vi "Instrument.DAQ.TestLauncher.vi"() -> ()   [LabVIEW 2019, in "Instrument.Lockin.lvlib" / "Instrument.DAQ.lvclass"]
uses:
  Instrument.DAQ.lvclass
  <vilib>/JKI/JKI SMO/SMO/Typedefs/SMOState --Enum.ctl
  Typedefs/AO.Channel--Cluster--Array.ctl
  Typedefs/AO.Channel--Cluster.ctl
  Typedefs/AO.Channel.Function--Enum.ctl
  Typedefs/REF.Channel--Cluster--Array.ctl
  Typedefs/REF.Channel--Cluster.ctl
  Typedefs/DAQ.Sampling.Sampling--Cluster.ctl
  Typedefs/Channel.Gain--Cluster--Array.ctl
  Typedefs/Channel.Gain--Cluster.ctl
  Typedefs/Status--enum.ctl
  Typedefs/DAQ.Configuration--Cluster.ctl
  Typedefs/DAQ.Config.AO.Range--enum.ctl
  Typedefs/DAQ.TerminalConfiguration--ring.ctl
  Typedefs/DAQ.Config.AI.Range--enum.ctl
  Typedefs/DAQ.Config.AI.Coupling--enum.ctl
  C:/Program Files/National Instruments/LabVIEW 2019/vi.lib/JKI/JKI SMO/SMO/SMO.lvclass
  <vilib>/JKI/JKI SMO/SMO/SMO.lvclass/SMO.ctl
  Typedefs/State--enum.ctl
  Typedefs/DAQ.Sampling--Cluster.ctl
  Instrument.Lockin/Typedefs/Results Type--Enum.ctl
  <vilib>/JKI/JKI SMO/SMO/Private/ReftoDVR--SMO.vi
  Instrument.Lockin/Instrument.Lockin.lvclass
  <vilib>/JKI/JKI SMO/SMO/SMO.lvclass
panel:
  out "DAQ state":T1
  in  "Tab Control 2":T2(tab)
  out "AO":waveform(dbl)[](graph)=[{"t0"=timestamp(3826459409.893437 s since 1904-01-01), "dt"=4.8830747732362694e-06, "Y"=array[15753 elements], "attributes"=variant("AO Channel"=variant(i32 1))}, {"t0"=timestamp(3826459409.893437 s since 1904-01-01), "dt"=4.8830747732362694e-06, "Y"=array[15753 elements], "attributes"=variant("AO Channel"=variant(i32 2))}, {"t0"=timestamp(3826459409.893437 s since 1904-01-01), "dt"=4.8830747732362694e-06, "Y"=array[15753 elements], "attributes"=variant("AO Channel"=variant(i32 3))}, {"t0"=timestamp(3826459409.893437 s since 1904-01-01), "dt"=4.8830747732362694e-06, "Y"=array[15753 elements], "attributes"=variant("AO Channel"=variant(i32 4))}]
  out "AI":waveform(dbl)[](graph)=[{"t0"=timestamp(3826459409.8699865 s since 1904-01-01), "dt"=4.883074773236228e-06, "Y"=array[15753 elements], "attributes"=variant("AI Channel"=variant(i32 1), "NI_ChannelName"=variant(string "PXI1Slot2/ai0"), "NI_UnitDescription"=variant(string "Volts"))}, {"t0"=timestamp(3826459409.8699865 s since 1904-01-01), "dt"=4.883074773236228e-06, "Y"=array[15753 elements], "attributes"=variant("AI Channel"=variant(i32 2), "NI_ChannelName"=variant(string "PXI1Slot2/ai1"), "NI_UnitDescription"=variant(string "Volts"))}, {"t0"=timestamp(3826459409.860074 s since 1904-01-01), "dt"=4.883074773236228e-06, "Y"=array[15753 elements], "attributes"=variant("AI Channel"=variant(i32 3), "NI_ChannelName"=variant(string "PXI1Slot3/ai0"), "NI_UnitDescription"=variant(string "Volts"))}, {"t0"=timestamp(3826459409.860074 s since 1904-01-01), "dt"=4.883074773236228e-06, "Y"=array[15753 elements], "attributes"=variant("AI Channel"=variant(i32 4), "NI_ChannelName"=variant(string "PXI1Slot3/ai1"), "NI_UnitDescription"=variant(string "Volts"))}]
  out "WFM 3":waveform(dbl)[](graph)=[{"t0"=timestamp(3826459409.893437 s since 1904-01-01), "dt"=4.8830747732362694e-06, "Y"=array[15753 elements], "attributes"=variant("AO Channel"=variant(i32 1))}, {"t0"=timestamp(3826459409.893437 s since 1904-01-01), "dt"=4.8830747732362694e-06, "Y"=array[15753 elements], "attributes"=variant("Reference Channel"=variant(i32 1))}, {"t0"=timestamp(3826459409.8699865 s since 1904-01-01), "dt"=4.883074773236228e-06, "Y"=array[15753 elements], "attributes"=variant("AI Channel"=variant(i32 1), "NI_ChannelName"=variant(string "PXI1Slot2/ai0"), "NI_UnitDescription"=variant(string "Volts"))}]
  out "REF":waveform(dbl)[](graph)=[{"t0"=timestamp(3826459409.893437 s since 1904-01-01), "dt"=4.8830747732362694e-06, "Y"=array[15753 elements], "attributes"=variant("Reference Channel"=variant(i32 1))}, {"t0"=timestamp(3826459409.893437 s since 1904-01-01), "dt"=4.8830747732362694e-06, "Y"=array[15753 elements], "attributes"=variant("Reference Channel"=variant(i32 1))}]
  out "Results":dbl[](graph)
  in  "Reset DAQ":bool
  in  "Stop DAQ":bool
  in  "Start DAQ":bool
  in  "Tab Control":enum32{"Output", "REF", "DAQ"}(tab)=enum."DAQ"
  in  "Channels: AO":T3=[{"Enable?"=TRUE, "Channel"=0, "Amplitude"=0.1, "Offset"=0.0, "Frequency"=15.0, "Phase"=0.0, "Function"=enum."sine", "Sweeping?"=FALSE, "Limit AC"=FALSE, "Limit DC?"=FALSE, "Duty Cycle"=FALSE}, {"Enable?"=TRUE, "Channel"=0, "Amplitude"=0.05, "Offset"=0.0, "Frequency"=13.0, "Phase"=0.0, "Function"=enum."sine", "Sweeping?"=FALSE, "Limit AC"=FALSE, "Limit DC?"=FALSE, "Duty Cycle"=FALSE}] {"Phase" format="%#_3g"; "Frequency" min=0.0001 max=200000.0 format="%#_6p"; "Offset" format="%#_6p"; "Amplitude" min=0.0 max=10.0 format="%#_6p"}
  in  "Channels: Lockin":T6=[{"Enable?"=TRUE, "Channel"=1, "Frequency"=13.0, "Phase"=0.0, "TC"=1e-05, "Roll-Off"=1}] {"Roll-Off" min=1 max=4; "TC" min=1e-06 max=100.0 format="%#_3p"; "Phase" format="%#_3p"; "Frequency" min=1e-06 max=102400.0 format="%#_6p"; "Channel" min=1}
  in  "Gain":T8
  in  "sampling":T10={"Fs"=204789.0, "#s"=15753} {"Fs" format="%#_13g"}
  in  "New Ch []":T11[](array[typedef])=[{"Device"="PXI1Slot2", "Lockin.AO"="", "AO.Ch"="", "AO.Range"=enum."±0.1", "AO terminal config"=0, "Lockin.AI"="", "AI.Ch"="", "AI.Range"=enum."±0.316", "AI.Coupling"=10050, "AI terminal config"=0}, {"Device"="PXI1Slot3", "Lockin.AO"="", "AO.Ch"="", "AO.Range"=enum."±0.1", "AO terminal config"=0, "Lockin.AI"="", "AI.Ch"="", "AI.Range"=enum."±0.316", "AI.Coupling"=10050, "AI terminal config"=0}] {"AI terminal config" items=[""=-1, "differential"=10106, "pseudodifferential"=12529]; "AI.Coupling" items=[""=0, "AC"=10045, "DC"=10050, "GND"=10066]; "AO terminal config" items=[""=-1, "differential"=10106, "pseudodifferential"=12529]}
  out "SMO State":T16=enum."Stopped"
  out "error out":errorcluster
  in  "Stop":bool
  # "Basic SMO Test Launcher"
  # "For instructions on how to use the JKI State Machine Objects, examples and video tutorials, visit:\nhttp://jki.net/state-machine-objects/\n\nJKI State Machine Objects™\nhttp://jki.net/state-machine-objects/\nCopyright (C) 2005-2015, JKI <info@jki.net>\nALL RIGHTS RESERVED"
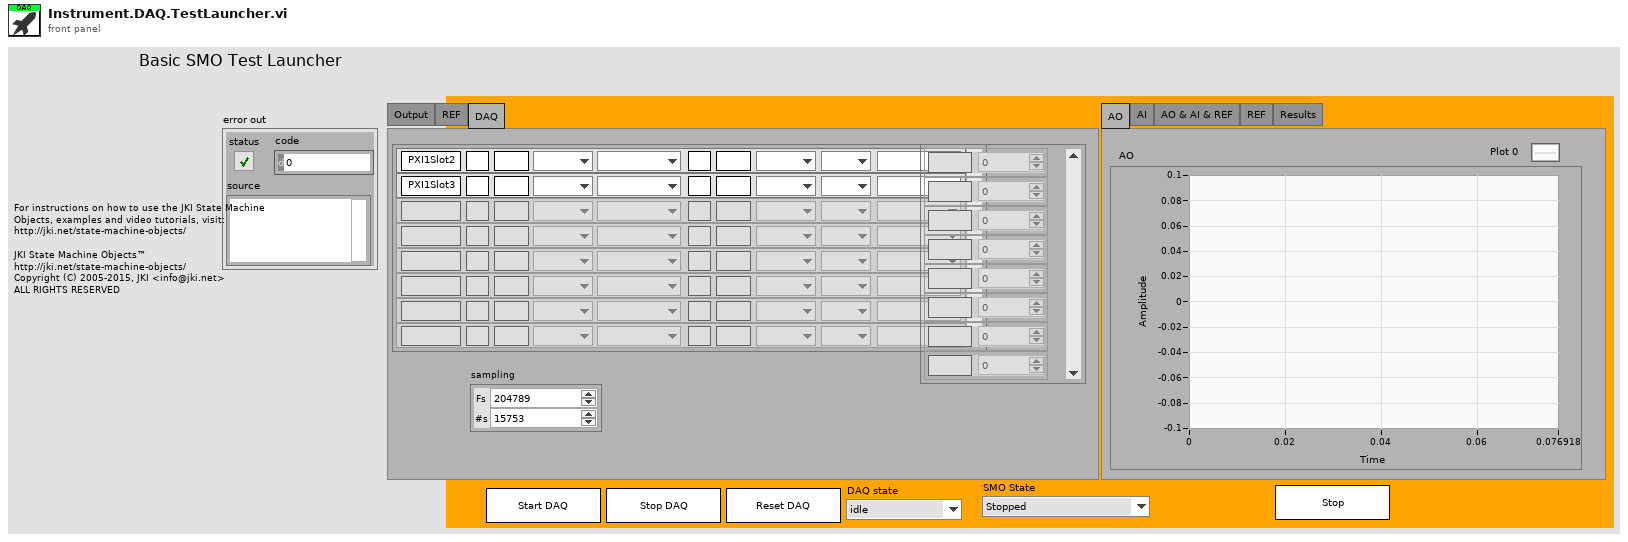
[diagram p1: front panel]
types:
  T1 = typedef "Instrument.Lockin.lvlib/Instrument.DAQ.lvclass/Status--enum.ctl" = enum16{"idle", "created", "started", "stopped", "sweeping"}
  T2 = enum32{"AO", "AI", "AO & AI & REF", "REF", "Results"}
  T3 = typedef "Instrument.Lockin.lvlib/Instrument.DAQ.lvclass/AO.Channel--Cluster--Array.ctl" = T4[]
  T4 = typedef "Instrument.Lockin.lvlib/Instrument.DAQ.lvclass/AO.Channel--Cluster.ctl" = cluster{"Enable?":bool, "Channel":i32, "Amplitude":dbl, "Offset":dbl, "Frequency":dbl, "Phase":dbl, "Function":T5, "Sweeping?":bool, "Limit AC":bool, "Limit DC?":bool, "Duty Cycle":bool}
  T5 = typedef "Instrument.Lockin.lvlib/Instrument.DAQ.lvclass/AO.Channel.Function--Enum.ctl" = enum16{"sine", "square", "triangle", "saw"}
  T6 = typedef "Instrument.Lockin.lvlib/Instrument.DAQ.lvclass/REF.Channel--Cluster--Array.ctl" = T7[]
  T7 = typedef "Instrument.Lockin.lvlib/Instrument.DAQ.lvclass/REF.Channel--Cluster.ctl" = cluster{"Enable?":bool, "Channel":i32, "Frequency":dbl, "Phase":dbl, "TC":dbl, "Roll-Off":i32}
  T8 = typedef "Instrument.Lockin.lvlib/Instrument.DAQ.lvclass/Channel.Gain--Cluster--Array.ctl" = T9[]
  T9 = typedef "Instrument.Lockin.lvlib/Instrument.DAQ.lvclass/Channel.Gain--Cluster.ctl" = cluster{"Channel":string, "Gain":dbl}
  T10 = typedef "Instrument.Lockin.lvlib/Instrument.DAQ.lvclass/DAQ.Sampling.Sampling--Cluster.ctl" = cluster{"Fs":dbl, "#s":i32}
  T11 = typedef "Instrument.Lockin.lvlib/Instrument.DAQ.lvclass/DAQ.Configuration--Cluster.ctl" = cluster{"Device":string, "Lockin.AO":string, "AO.Ch":string, "AO.Range":T12, "AO terminal config":T13, "Lockin.AI":string, "AI.Ch":string, "AI.Range":T14, "AI.Coupling":T15, "AI terminal config":T13}
  T12 = typedef "Instrument.Lockin.lvlib/Instrument.DAQ.lvclass/DAQ.Config.AO.Range--enum.ctl" = enum16{"±0.1", "±1.0", "±3.5", "±10.0", ""}
  T13 = typedef "Instrument.Lockin.lvlib/Instrument.DAQ.lvclass/DAQ.TerminalConfiguration--ring.ctl" = i32
  T14 = typedef "Instrument.Lockin.lvlib/Instrument.DAQ.lvclass/DAQ.Config.AI.Range--enum.ctl" = enum16{"±0.316", "±1.00", "±3.16", "±10.0", "±31.6", "±42.4", ""}
  T15 = typedef "Instrument.Lockin.lvlib/Instrument.DAQ.lvclass/DAQ.Config.AI.Coupling--enum.ctl" = u16
  T16 = typedef "SMO.lvclass/SMOState --Enum.ctl" = enum16{"unknown", "Created", "Started", "Stopped"}
  T17 = typedef "SMO.lvclass/Public Events.ctl" = cluster{"Error":refnum<user-event>, "State":refnum<user-event>, "Reserve State":refnum<user-event>}
  T18 = typedef "Instrument.Lockin.lvlib/Instrument.DAQ.lvclass/PublicEvents--Cluster.ctl" = cluster{"getAIChannels":refnum<user-event>, "getAOChannels":refnum<user-event>, "getREFChannels":refnum<user-event>, "getWaveforms":refnum<user-event>, "getResults":refnum<user-event>, "getSweepWaveforms":refnum<user-event>, "getCalibration":refnum<user-event>, "getDAQState":refnum<user-event>, "getDAQconfig":refnum<user-event>, "getInputGain":refnum<user-event>, "getOutputGain":refnum<user-event>, "getInputOffset":refnum<user-event>, "getSampling":refnum<user-event>, "getSweepChannels":refnum<user-event>, "getDeviceIDN":refnum<user-event>}
  T19 = cluster{"Event Registration Refnum":refnum<event-registration>}
  T20 = typedef "Instrument.Lockin.lvlib/Instrument.DAQ.lvclass/State--enum.ctl" = enum16{"start", "stop", "reset", "start sweep", "stop sweep"}
  T21 = typedef "Instrument.Lockin.lvlib/Instrument.DAQ.lvclass/DAQ.Sampling--Cluster.ctl" = cluster{"Sampling":T10, "Fs_Out":dbl}
  T22 = typedef "Instrument.Lockin.lvlib/Instrument.Lockin.lvclass/Results Type--Enum.ctl" = enum16{"X", "Y", "R", "Theta", "Mean"}
  T23 = typedef "Instrument.Lockin.lvlib/Instrument.DAQ.lvclass/DAQ.Config.AO--Cluster--Array.ctl" = cluster{"Channels":tag, "Range":T12, "terminal configuration":T13, "Type":T24}[]
  T24 = typedef "Instrument.Lockin.lvlib/Instrument.DAQ.lvclass/DAQ.Type--enum.ctl" = enum16{"None", "USB-4431", "PXI-446x"}
  T25 = typedef "Instrument.Lockin.lvlib/Instrument.DAQ.lvclass/DAQ.Config.AI--Cluster--Array.ctl" = cluster{"Channels":tag, "Coupling":T15, "Range":T14, "terminal configuration":T13, "Type":T24}[]
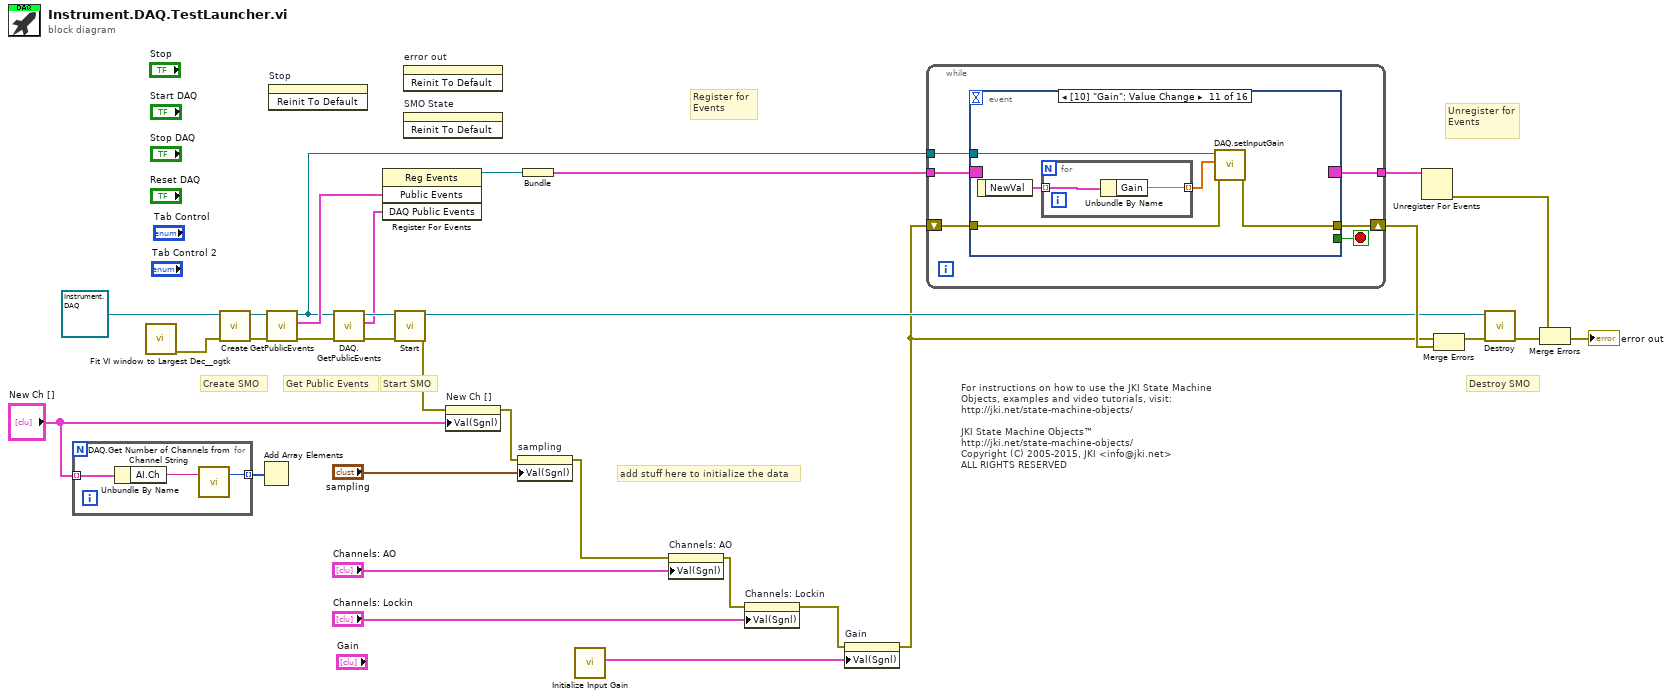
[diagram p0: block diagram]
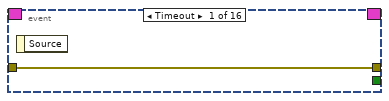
[diagram p2: hidden frame]
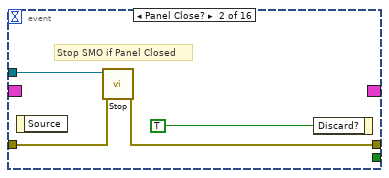
[diagram p3: hidden frame]
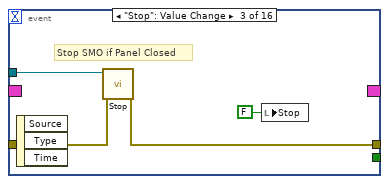
[diagram p4: hidden frame]
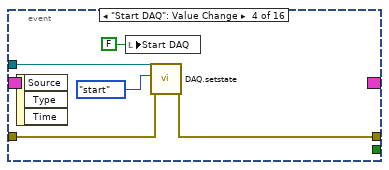
[diagram p5: hidden frame]
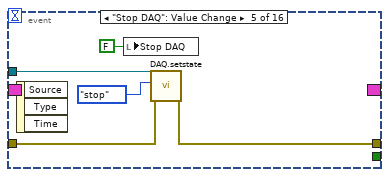
[diagram p6: hidden frame]
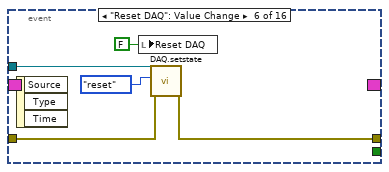
[diagram p7: hidden frame]
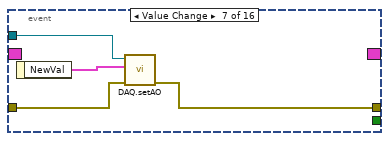
[diagram p8: hidden frame]
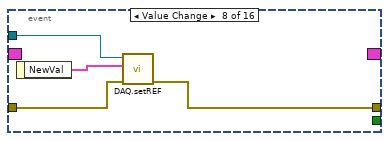
[diagram p9: hidden frame]
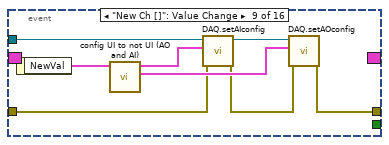
[diagram p10: hidden frame]
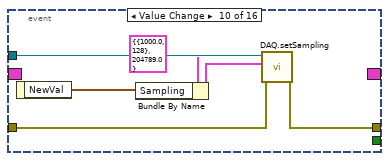
[diagram p11: hidden frame]
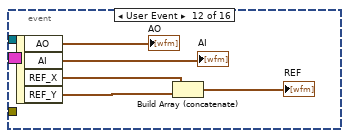
[diagram p12: hidden frame]
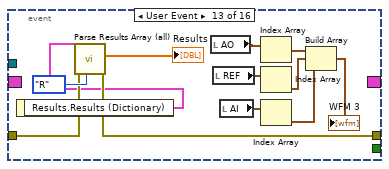
[diagram p13: hidden frame]
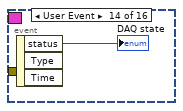
[diagram p14: hidden frame]
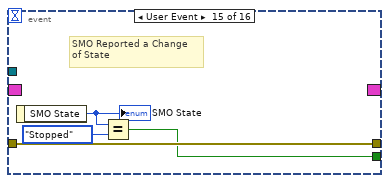
[diagram p15: hidden frame]
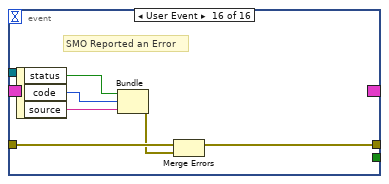
[diagram p16: hidden frame]
diagram:
  # "add stuff here to initialize the data"
  # "For instructions on how to use the JKI State Machine Objects, examples and video tutorials, visit:\nhttp://jki.net/state-machine-objects/\n\nJKI State Machine Objects™\nhttp://jki.net/state-machine-objects/\nCopyright (C) 2005-2015, JKI <info@jki.net>\nALL RIGHTS RESERVED"
  # "Get Public Events"
  # "Start SMO"
  # "Destroy SMO"
  # "Create SMO"
  # "Unregister for Events"
  # "Register for Events"
  n1 = for {
    tunnel: "New Ch []" -> [w34] mode=indexing
    tunnel: [w33] -> w10 mode=indexing
    n2 = Unbundle By Name(w34) -> ("AI.Ch"=w32:string)
    n3 = call "DAQ.Get Number of Channels from Channel String.vi"("Channels String"=w32) -> ("# channels"=w33:i32)  [unwired: 2 in]
  }
  n4 = call <userlib>:"Fit VI window to Largest Dec__ogtk.vi"() -> ("error out"=w7:errorcluster)  [unwired: 6 in, 1 out]
  n5 = call <vilib>:"Create.vi"("error in (no error)"=w7, "SMO"=refnum<class "Instrument.DAQ.lvclass"> refnum ("Lockin.DAQ.lvclass")) -> ("error out"=w23:errorcluster, "SMO out"=w24:refnum<class "Instrument.DAQ.lvclass">)  [unwired: 7 in, 1 out]
  n6 = Add Array Elements(numeric array=w10) -> ()  [unwired: 1 out]
  n7 = call <vilib>:"GetPublicEvents.vi"("error in (no error)"=w23, "SMO"=w24) -> ("error out"=w20:errorcluster, "Public Events"=w22:T17, "SMO out"=w19:refnum<class "Instrument.DAQ.lvclass">)  [unwired: 7 in]
  n8 = invoke on="Stop" class="Bool (strict)" method="Reinit To Default"() -> ()  [unwired: 3 in, 3 out]
  n9 = call "DAQ.GetPublicEvents.vi"("error in (no error)"=w20, "Instrument.DAQ"=w19) -> ("error out"=w17:errorcluster, "DAQ Public Events"=w16:T18, "Instrument.DAQ out"=w18:refnum<class "Instrument.DAQ.lvclass">)  [unwired: 7 in]
  n10 = register-events(w22, w16) -> (reference out=w21:refnum<event-registration>)  [unwired: 2 in, 1 out]
  n11 = call <vilib>:"Start.vi"("error in (no error)"=w17, "SMO"=w18) -> ("error out"=w4:errorcluster, "SMO out"=w11:refnum<class "Instrument.DAQ.lvclass">)  [unwired: 8 in]
  n12 = invoke on="error out" class="Clust (strict)" method="Reinit To Default"() -> ()  [unwired: 3 in, 3 out]
  n13 = invoke on="SMO State" class="Enum (strict)" method="Reinit To Default"() -> ()  [unwired: 3 in, 3 out]
  n14 = property on="New Ch []" class="Arr (strict)"(error in=w4, "Val(Sgnl)"="New Ch []") -> (error out=w3:errorcluster)  [unwired: 1 in, 1 out]
  n15 = property on="sampling" class="Clust (strict)"(error in=w3, "Val(Sgnl)"="sampling") -> (error out=w2:errorcluster)  [unwired: 1 in, 1 out]
  n16 = Bundle("Event Registration Refnum"=w21) -> (w30:T19)  [unwired: 1 in]
  n17 = call "Initialize Input Gain.vi"() -> ("Input Gain"=w1:T8)  [unwired: 9 in, 2 out]
  n18 = property on="Channels: AO" class="Arr (strict)"(error in=w2, "Val(Sgnl)"="Channels: AO") -> (error out=w12:errorcluster)  [unwired: 1 in, 1 out]
  n19 = property on="Channels: Lockin" class="Arr (strict)"(error in=w12, "Val(Sgnl)"="Channels: Lockin") -> (error out=w9:errorcluster)  [unwired: 1 in, 1 out]
  n20 = property on="Gain" class="Arr (strict)"(error in=w9, "Val(Sgnl)"=w1) -> (error out=w6:errorcluster)  [unwired: 1 in, 1 out]
  n21 = while {
    shift-right: [w39] -> w29
    shift-left: w6 -> [w38]
    tunnel: w30 -> [w37]
    tunnel: [w36] -> w31
    tunnel: w19 -> [w35]
    stop <- w40 stop-if-true
    n22 = event shown="[10] \"Gain\": Value Change" {
      selector: w37 -> [_ _ _ _ _ _ _ _ _ _ _ _ _ _ _ _]
      dyn-events: [_ _ _ _ _ _ _ _ _ _ _ _ _ _ _ _] -> w36
      timeout: _ -> [_ _ _ _ _ _ _ _ _ _ _ _ _ _ _ _]
      tunnel: [_ _ _ _ _ _ _ _ _ _ _ _ _ _ w112 _] -> w40
      tunnel: w35 -> [_ w45 w49 w54 w59 w64 w67 w71 w75 w86 w91 _ _ _ _ _]
      tunnel: [w41 w44 w48 w53 w58 w63 w65 w69 w80 w84 w89 _ w101 _ w115 w119] -> w39
      tunnel: w38 -> [w41 w43 w47 w52 w57 w62 w66 w70 w73 w85 w90 _ w102 _ w115 w117]
      event Timeout {
        n23 = event-data() -> ()  [unwired: 1 in, 1 out]
      }
      event Panel Close? {
        # "Stop SMO if Panel Closed"
        n24 = event-data() -> ()  [unwired: 1 in, 1 out]
        n25 = call <vilib>:"Stop.vi"("error in (no error)"=w43, "SMO"=w45) -> ("error out"=w44:errorcluster)  [unwired: 8 in, 1 out]
        n26 = event-data("Discard?"=TRUE ("OK")) -> ()  [unwired: 1 in, 1 out]
      }
      event "Stop": Value Change {
        # "Stop SMO if Panel Closed"
        n27 = event-data() -> ()  [unwired: 1 in, 3 out]
        n28 = call <vilib>:"Stop.vi"("error in (no error)"=w47, "SMO"=w49) -> ("error out"=w48:errorcluster)  [unwired: 8 in, 1 out]
        n29 = local write "Stop"(FALSE ("Stop")) -> ()
      }
      event "Start DAQ": Value Change {
        n30 = event-data() -> ()  [unwired: 1 in, 3 out]
        n31 = local write "Start DAQ"(FALSE ("Start DAQ")) -> ()
        n32 = call "DAQ.setstate.vi"("error in (no error)"=w52, "setState"=State--enum."start", "Instrument.DAQ"=w54) -> ("error out"=w53:errorcluster)  [unwired: 7 in, 1 out]
      }
      event "Stop DAQ": Value Change {
        n33 = event-data() -> ()  [unwired: 1 in, 3 out]
        n34 = local write "Stop DAQ"(FALSE ("Stop DAQ")) -> ()
        n35 = call "DAQ.setstate.vi"("error in (no error)"=w57, "setState"=State--enum."stop", "Instrument.DAQ"=w59) -> ("error out"=w58:errorcluster)  [unwired: 7 in, 1 out]
      }
      event "Reset DAQ": Value Change {
        n36 = event-data() -> ()  [unwired: 1 in, 3 out]
        n37 = local write "Reset DAQ"(FALSE ("Reset DAQ")) -> ()
        n38 = call "DAQ.setstate.vi"("error in (no error)"=w62, "setState"=State--enum."reset", "Instrument.DAQ"=w64) -> ("error out"=w63:errorcluster)  [unwired: 7 in, 1 out]
      }
      event Value Change {
        n39 = event-data() -> ("NewVal"=w68:T3)  [unwired: 1 in]
        n40 = call "DAQ.setAO.vi"("error in (no error)"=w66, "AO Channels"=w68, "Instrument.DAQ"=w67) -> ("error out"=w65:errorcluster)  [unwired: 7 in, 1 out]
      }
      event Value Change {
        n41 = event-data() -> ("NewVal"=w72:T6)  [unwired: 1 in]
        n42 = call "DAQ.setREF.vi"("error in (no error)"=w70, "Channels: Lockin"=w72, "Instrument.DAQ"=w71) -> ("error out"=w69:errorcluster)  [unwired: 7 in, 1 out]
      }
      event "New Ch []": Value Change {
        n43 = event-data() -> ("NewVal"=w79:T11[])  [unwired: 1 in]
        n44 = call "config UI to not UI (AO and AI).vi"("New Ch []"=w79) -> ("AO Config"=w77:T23, "AI Config"=w78:T25)  [unwired: 9 in]
        n45 = call "DAQ.setAIconfig.vi"("error in (no error)"=w73, "AI Configuration"=w78, "Instrument.DAQ"=w75) -> ("error out"=w74:errorcluster, "Instrument.DAQ out"=w76:refnum<class "Instrument.DAQ.lvclass">)  [unwired: 7 in]
        n46 = call "DAQ.setAOconfig.vi"("error in (no error)"=w74, "AO Configuration"=w77, "Instrument.DAQ"=w76) -> ("error out"=w80:errorcluster)  [unwired: 7 in, 1 out]
      }
      event Value Change {
        n47 = event-data() -> ("NewVal"=w82:T10)  [unwired: 1 in]
        n48 = Bundle By Name(cluster=T21 {"Sampling"={"Fs"=1000.0, "#s"=128}, "Fs_Out"=204789.0} ("Sampling"), "Sampling"=w82) -> (w81:T21)
        n49 = call "DAQ.setSampling.vi"("error in (no error)"=w85, "Sampling"=w81, "Instrument.DAQ"=w86) -> ("error out"=w84:errorcluster)  [unwired: 7 in, 1 out]
      }
      event Value Change {
        n50 = event-data() -> ("NewVal"=w88:T8)  [unwired: 1 in]
        n51 = for {
          tunnel: w88 -> [w93] mode=indexing
          tunnel: [w92] -> w87 mode=indexing
          n52 = Unbundle By Name(w93) -> ("Gain"=w92:dbl)
        }
        n53 = call "DAQ.setInputGain.vi"("error in (no error)"=w90, "Input Gain"=w87, "Instrument.DAQ"=w91) -> ("error out"=w89:errorcluster)  [unwired: 7 in, 1 out]
      }
      event User Event {
        n54 = event-data() -> ("AO"=→"AO":waveform(dbl)[], "AI"=→"AI":waveform(dbl)[], "REF_X"=w96:waveform(dbl)[], "REF_Y"=w95:waveform(dbl)[])  [unwired: 1 in]
        n55 = Build Array (concatenate)(w96, w95) -> (→"REF":waveform(dbl)[])
      }
      event User Event {
        n56 = event-data() -> ("Results.Results (Dictionary)"=w99:cluster{"key":string, "value":dbl[]}[])  [unwired: 1 in]
        n57 = call "Parse Results Array (all).vi"("Type"=Results_Type--Enum."R", "error in (no error)"=w102, "Results (Dictionary)"=w99) -> ("error out"=w101:errorcluster, "Data"=→"Results":dbl[])  [unwired: 5 in, 2 out]
        n58 = local read "AO"() -> (w110:waveform(dbl)[])
        n59 = local read "REF"() -> (w109:waveform(dbl)[])
        n60 = local read "AI"() -> (w108:waveform(dbl)[])
        n61 = Index Array(array=w110) -> (element=w107:waveform(dbl))  [unwired: 1 in]
        n62 = Index Array(array=w109) -> (element=w106:waveform(dbl))  [unwired: 1 in]
        n63 = Index Array(array=w108) -> (element=w104:waveform(dbl))  [unwired: 1 in]
        n64 = Build Array(w107, w106, w104) -> (→"WFM 3":waveform(dbl)[])
      }
      event User Event {
        n65 = event-data() -> ("status"=→"DAQ state":T1)  [unwired: 1 in, 2 out]
      }
      event User Event {
        # "SMO Reported a Change\nof State"
        n66 = event-data() -> ("SMO State"=w114:T16)  [unwired: 1 in]
        "SMO State" <- w114
        n67 = Equal?(x=w114, y=SMOState_--Enum."Stopped") -> (x = y?=w112:bool)
      }
      event User Event {
        # "SMO Reported an Error"
        n68 = event-data() -> ("status"=w118:bool, "code"=w121:i32, "source"=w120:string)  [unwired: 1 in]
        n69 = Bundle("status"=w118, "code"=w121, "source"=w120) -> (w116:errorcluster)  [unwired: 1 in]
        n70 = Merge Errors(w117, w116) -> (w119:errorcluster)
      }
    }
  }
  n71 = Unregister For Events(event registration refnum=w31) -> (error out=w28:errorcluster)  [unwired: 1 in]
  n72 = Merge Errors(w6, w29) -> (w25:errorcluster)
  n73 = call <vilib>:"Destroy.vi"("error in (no error)"=w25, "SMO"=w11) -> ("error out"=w26:errorcluster)  [unwired: 9 in]
  n74 = Merge Errors(w28, w26) -> (→"error out":errorcluster)
